vi "Begin.vi"() -> (0 "error out":errorcluster)   [LabVIEW 2013]
doc: "Called before other user functions, this VI is expected to open initial I/O refnums, load in file data, and do all program initialization. Notice that the <B>error out</B> terminal is simply used for data flow. Wiring it to other structures or subVIs ensures that this VI runs first."
uses:
  <vilib>/Rock Robotics/WPI/DriverStation/WPI_DriverStationRobotMode2.ctl
  <vilib>/Rock Robotics/WPI/Solenoid/WPI_SolenoidChannel.ctl
  <vilib>/Rock Robotics/WPI/SafetyOutput/WPI_SafetyOutputConfigMenu.ctl
  <vilib>/Rock Robotics/SystemInterfaces/DIO/FPGA_DIOChannel.ctl
  <vilib>/Rock Robotics/SystemInterfaces/DIO/FPGA_DIORelayChannel.ctl
  <vilib>/Rock Robotics/SystemInterfaces/AI/FPGA_AIGyroChannel.ctl
  <vilib>/Rock Robotics/SystemInterfaces/DIO/FPGA_DIOPWMChannel.ctl
  <vilib>/Rock Robotics/WPI/Joystick/WPI_JoystickDeviceEnum.ctl
  Robot Global Data.vi
  <vilib>/Rock Robotics/WPI/Solenoid/WPI_SolenoidOpenDouble.vi
  <vilib>/Rock Robotics/WPI/Counter/WPI_CounterDigitalInputToDigitalSource.vi
  <vilib>/Rock Robotics/WPI/MotorControl/WPI_MotorControlOpen Talon.vi
  <vilib>/Rock Robotics/WPI/Counter/WPI_CounterOpen Semi Period Mode.vi
  Auto Pickup Global.vi
  <vilib>/Rock Robotics/WPI/Compressor/WPI_CompressorGetSetRefNum.vi
  <vilib>/Rock Robotics/WPI/Relay/WPI_RelayDirection.ctl
  <vilib>/Rock Robotics/WPI/RobotDrive/WPI_RobotDriveOpen4MotorWithCANJaguar.vi
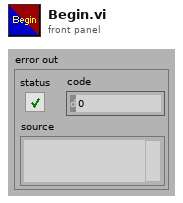
[diagram p1: front panel]
types:
  T1 = typedef "FPGA_DIOChannel.ctl" = enum8{"DIO 1", "DIO 2", "DIO 3", "DIO 4", "DIO 5", "DIO 6", "DIO 7", "DIO 8", "DIO 9", "DIO 10", "DIO 11", "DIO 12", "DIO 13", "DIO 14", "Invalid"}
  T2 = typedef "FPGA_DIOPWMChannel.ctl" = enum8{"PWM 1", "PWM 2", "PWM 3", "PWM 4", "PWM 5", "PWM 6", "PWM 7", "PWM 8", "PWM 9", "PWM 10", "Invalid"}
  T3 = typedef "WPI_JoystickDeviceEnum.ctl" = enum16{"USB 1", "USB 2", "USB 3", "USB 4", "Kinect 1", "Kinect 2"}
  T4 = typedef "WPI_SafetyOutputConfigMenu.ctl" = enum16{"Enable", "Disable"}
  T5 = typedef "FPGA_AIGyroChannel.ctl" = enum8{"AI 1", "AI 2", "Invalid"}
  T6 = typedef "FPGA_DIORelayChannel.ctl" = enum8{"Relay 1", "Relay 2", "Relay 3", "Relay 4", "Relay 5", "Relay 6", "Relay 7", "Relay 8", "Invalid"}
  T7 = typedef "WPI_SolenoidChannel.ctl" = enum8{"Solenoid 1", "Solenoid 2", "Solenoid 3", "Solenoid 4", "Solenoid 5", "Solenoid 6", "Solenoid 7", "Solenoid 8", "Invalid"}
  T8 = typedef "WPI_DriverStationRobotMode2.ctl" = enum16{"Autonomous Disabled", "Autonomous Enabled", "Teleop Disabled", "Teleop Enabled", "Timeout", "Finish", "Test Disabled", "Test Enabled"}
  T9 = typedef "WPI_RobotDriveDevRef.ctl" = cluster{"DevStatus":errorcluster, "Motors[]":T10[], "Square Inputs":bool, "Max Output":dbl, "Isochronous":bool}
  T10 = typedef "WPI_MotorControlDeviceRef.ctl" = cluster{"DeviceStatus":errorcluster, "Type":enum16{"PWM", "CAN"}, "PWM":cluster{"Digital Module":T11, "PWM Channel":T2, "DeadBand":T12}, "CAN":cluster{"Device Number":u8, "Control Mode":T13, "Semaphore":T14, "Max Vout":dbl}, "Invert":bool, "TransformRef":T15, "InvTransformRef":T15}
  T11 = typedef "FPGA_TypedefDigitalModule.ctl" = enum16{"Digital Module 1", "Digital Module 2"}
  T12 = typedef "WPI_PWMDeadband.ctl" = cluster{"Name":string, "maxPositivePwm":i32, "minPositivePwm":i32, "centerPwm":i32, "maxNegativePwm":i32, "minNegativePwm":i32, "angularRange":u16}
  T13 = typedef "WPI_CANJaguar_ControlMode.ctl" = enum8{"Percent VBus", "Current", "Speed", "Position", "Voltage"}
  T14 = typedef "Semaphore RefNum" = refnum<k1>
  T15 = typedef "WPI_PWMTransform_ConPane.ctl" = refnum<vi>
  T16 = typedef "WPI_DigitalInputDevRef.ctl" = cluster{"DevStatus":errorcluster, "DIO Channel":T1, "Digital Module":T11}
  T17 = typedef "FPGA_CounterEncoderSourceConvertionLVSourceType.ctl" = cluster{"DevStatus":errorcluster, "AnalogTriggerMode?":bool, "DigitalMode":cluster{"Digital Module":T11, "DIO Channel":T18}, "AnalogTriggerMode":cluster{"AnalogTriggerIndex":T19, "OutputType":T20}}
  T18 = typedef "FPGA_DIODigitalSourceChannel.ctl" = enum8{"DIO 1", "DIO 2", "DIO 3", "DIO 4", "DIO 5", "DIO 6", "DIO 7", "DIO 8", "DIO 9", "DIO 10", "DIO 11", "DIO 12", "DIO 13", "DIO 14", "Disabled"}
  T19 = typedef "FPGA_AnalogTriggerIndex.ctl" = enum8{"Trig 0", "Trig 1", "Trig 2", "Trig 3", "Trig 4", "Trig 5", "Trig 6", "Trig 7", "Invalid"}
  T20 = typedef "FPGA_AnalogTriggerOutType.ctl" = enum16{"InWindow", "TriggerState", "Rising", "Falling"}
  T21 = typedef "WPI_CompressorDevRef.ctl" = cluster{"DevStatus":errorcluster, "DigitalInputDevRef":T16, "RelayDevRef":T22}
  T22 = typedef "WPI_RelayDevRef.ctl" = cluster{"DevStatus":errorcluster, "Relay Channel":T6, "Digital Module":T11, "Relay Direction":T23}
  T23 = typedef "WPI_RelayDirection.ctl" = enum16{"Both directions", "Forward only", "Reverse only"}
  T24 = typedef "WPI_EncoderDevRef.ctl" = cluster{"DevStatus":errorcluster, "EncoderIndex":T25, "CounterIndex":T26, "DistancePerCount":dbl, "Decoding Type":T27}
  T25 = typedef "FPGA_EncoderIdx.ctl" = enum8{"Enc 0", "Enc 1", "Enc 2", "Enc 3", "Invalid"}
  T26 = typedef "FPGA_CounterCtrSystemIndex.ctl" = enum8{"Ctr 0", "Ctr 1", "Ctr 2", "Ctr 3", "Ctr 4", "Ctr 5", "Ctr 6", "Ctr 7", "Invalid"}
  T27 = typedef "WPI_EncoderType.ctl" = enum16{"1x", "2x", "4x"}
  T28 = typedef "WPI_CounterDevRef.ctl" = cluster{"DevStatus":errorcluster, "CntIndex":T26}
  T29 = typedef "WPI_GyroDevRef.ctl" = cluster{"DevStatus":errorcluster, "Analog Module":T30, "Analog Channel":T31, "Offset":dbl, "Gain (VoltsPerDegree/Second)":dbl}
  T30 = typedef "FPGA_TypedefAnalogModule.ctl" = enum16{"Analog Module 1", "Analog Module 2"}
  T31 = typedef "FPGA_AIChannel.ctl" = enum8{"AI 1", "AI 2", "AI 3", "AI 4", "AI 5", "AI 6", "AI 7", "AI 8", "Invalid"}
  T32 = typedef "WPI_I2CDevRef.ctl" = cluster{"DevStatus":errorcluster, "Digital Module":T11, "Device Address":u8}
  T33 = typedef "WPI_JoystickDevRef.ctl" = cluster{"Device":T3}
  T34 = typedef "LEDStripRef.ctl" = cluster{"PWM Rate (Hz)":sgl, "Max Duty Cycle":sgl, "DigitalOutputRed":T35, "DigitalOutputGreen":T35, "DigitalOutputBlue":T35, "DevStatus":errorcluster}
  T35 = typedef "WPI_DigitalOutputDevRef.ctl" = cluster{"Digital Module":T11, "DIO Channel":T1, "DevStatus":errorcluster}
  T36 = typedef "WPI_SolenoidDevRef.ctl" = cluster{"DevStatus":errorcluster, "Solenoid Module":T37, "Forward Solenoid Channel":T7, "Reverse Solenoid Channel":T7}
  T37 = typedef "FPGA_TypedefSolenoidModule.ctl" = enum16{"Solenoid Module 1", "Solenoid Module 2"}
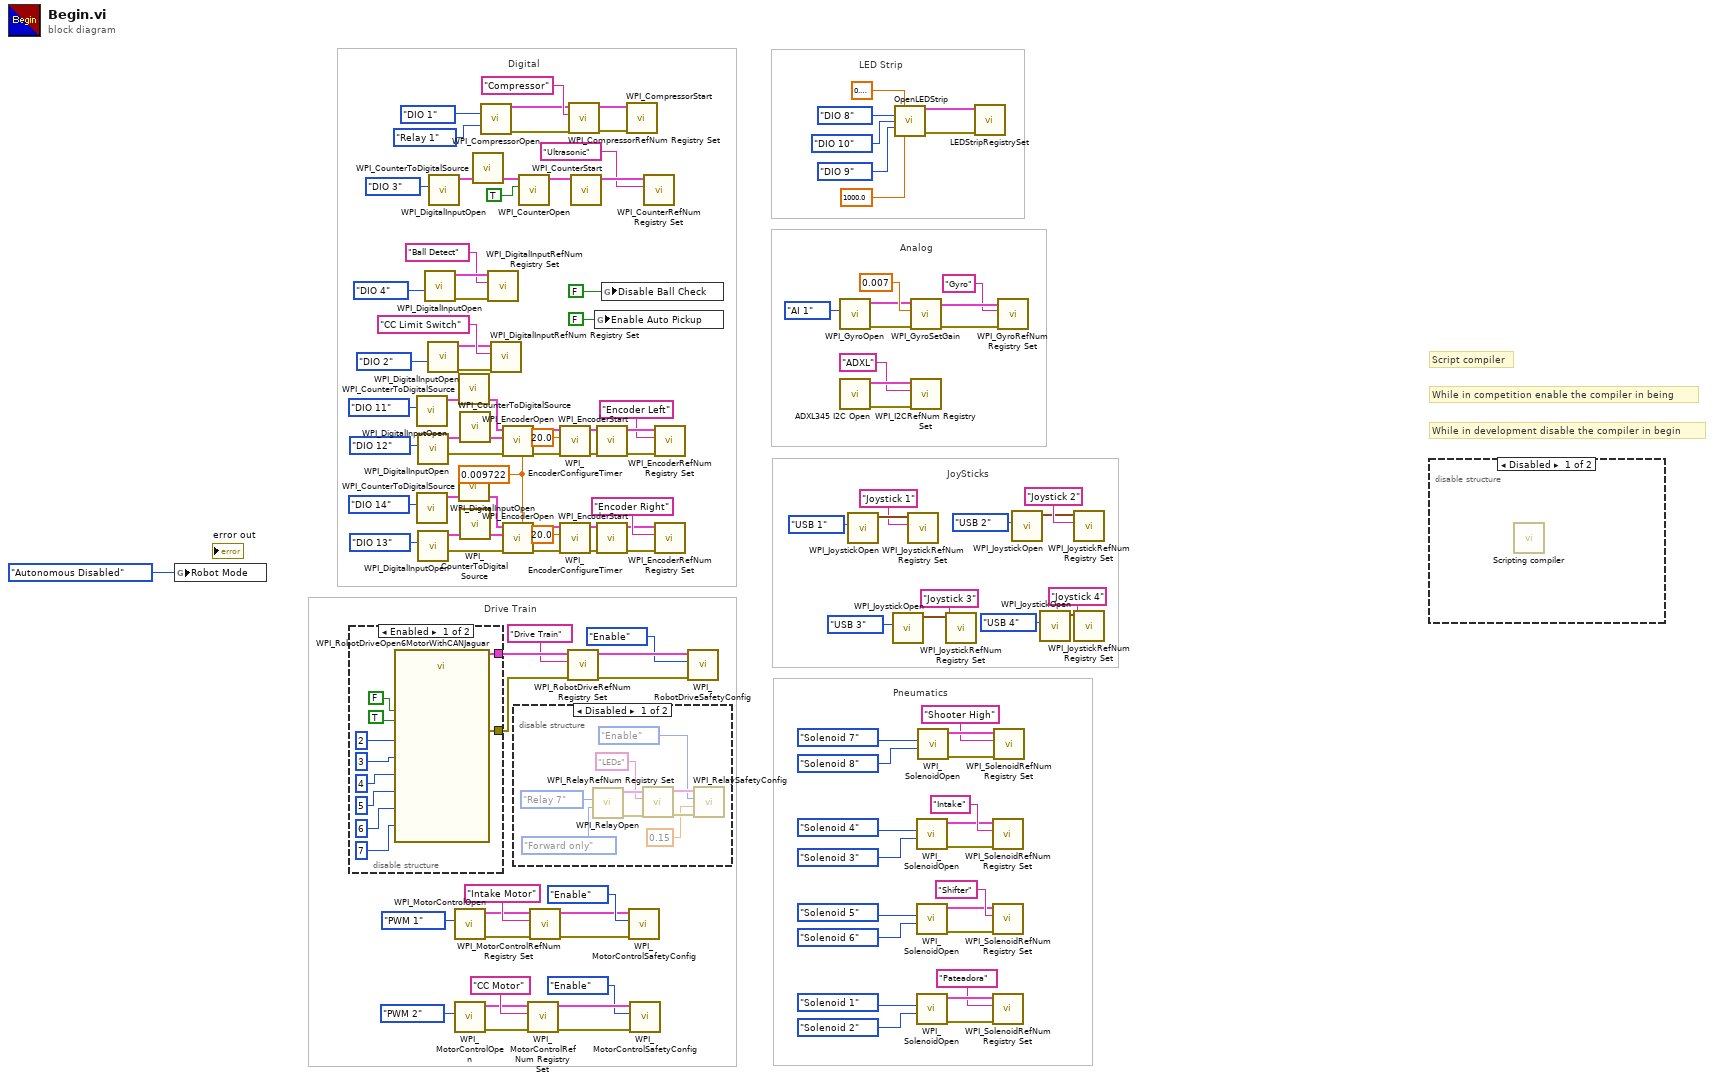
[diagram p0: block diagram]
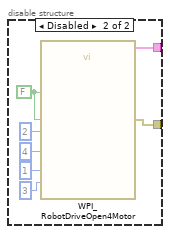
[diagram p3: hidden frame]
diagram:
  w11 = 0.009722 ("DistancePerCount")
  # "LED Strip"
  # "While in development disable the compiler in begin"
  # "While in competition enable the compiler in being"
  # "Script compiler"
  # "JoySticks"
  # "Analog"
  # "Digital"
  # "Drive Train"
  # "Pneumatics"
  n1 = global write "Robot Global Data.vi" "Robot Mode"(WPI_DriverStationRobotMode2."Autonomous Disabled" ("Robot Mode")) -> ()
  n2 = disable-structure shown="Enabled" {
    disable-tunnel: [w133 w142] -> w107
    disable-tunnel: [w132 w136] -> w100
    frame Enabled {
      n3 = call <vilib>:"WPI_RobotDriveOpen6MotorWithCANJaguar.vi"("Rear Left Motor"=u8 4, "Rear Right Motor"=u8 7 ("Mid Right Motor"), "Front Right Motor"=u8 5 ("Rear Right Motor"), "Front Left Motor"=u8 2, "Mid Left Motor"=u8 3 ("Front Right Motor"), "Mid Right Motor"=u8 6 ("Mid Left Motor"), "Left Motors Inverted"=FALSE, "Right Motors Inverted"=TRUE) -> ("RobotDriveDevRef"=w133:T9, "error out"=w132:errorcluster)  [unwired: 10 in]
    }
    frame Disabled {
      w137 = FALSE ("Front Left Motor Inverted")
      n4 = call-poly <vilib>:"WPI_RobotDriveOpen4Motor.vi"("Rear Left Motor"=u8 4, "Rear Left Motor Inverted"=w137, "Rear Right Motor"=u8 3, "Front Left Motor"=u8 2, "Front Right Motor"=u8 1, "Front Left Motor Inverted"=w137) -> ("RobotDriveDevRef"=w142:T9, "error out"=w136:errorcluster)  [unwired: 8 in]
    }
  }
  n5 = call <vilib>:"WPI_DigitalInputOpen.vi"("DIO Channel"=FPGA_DIOChannel."DIO 11") -> ("DigitalInputDevRef"=w99:T16)  [unwired: 2 in, 8 out]
  n6 = call <vilib>:"WPI_DigitalInputOpen.vi"("DIO Channel"=FPGA_DIOChannel."DIO 14") -> ("DigitalInputDevRef"=w14:T16)  [unwired: 2 in, 8 out]
  n7 = call <vilib>:"WPI_DigitalInputOpen.vi"("DIO Channel"=FPGA_DIOChannel."DIO 12") -> ("error out"=w85:errorcluster, "DigitalInputDevRef"=w90:T16)  [unwired: 2 in, 7 out]
  n8 = call <vilib>:"WPI_DigitalInputOpen.vi"("DIO Channel"=FPGA_DIOChannel."DIO 13") -> ("error out"=w28:errorcluster, "DigitalInputDevRef"=w23:T16)  [unwired: 2 in, 7 out]
  n9 = call <vilib>:"WPI_DigitalInputOpen.vi"("DIO Channel"=FPGA_DIOChannel."DIO 4") -> ("error out"=w29:errorcluster, "DigitalInputDevRef"=w32:T16)  [unwired: 9 in]
  n10 = call <vilib>:"WPI_DigitalInputOpen.vi"("DIO Channel"=FPGA_DIOChannel."DIO 2") -> ("error out"=w81:errorcluster, "DigitalInputDevRef"=w82:T16)  [unwired: 9 in]
  n11 = call <vilib>:"WPI_DigitalInputOpen.vi"("DIO Channel"=FPGA_DIOChannel."DIO 3") -> ("DigitalInputDevRef"=w43:T16)  [unwired: 2 in, 8 out]
  n12 = call-poly <vilib>:"WPI_MotorControlOpen.vi"("PWM Channel"=FPGA_DIOPWMChannel."PWM 1") -> ("error out"=w70:errorcluster, "MotorControlDeviceRef"=w62:T10)  [unwired: 9 in]
  n13 = call-poly <vilib>:"WPI_MotorControlOpen.vi"("PWM Channel"=FPGA_DIOPWMChannel."PWM 2") -> ("error out"=w67:errorcluster, "MotorControlDeviceRef"=w61:T10)  [unwired: 9 in]
  n14 = call-poly <vilib>:"WPI_CounterToDigitalSource.vi"("DigitalInputDevRef"=w99) -> ("Digital Source"=w98:T17)  [unwired: 6 out]
  n15 = call-poly <vilib>:"WPI_CounterToDigitalSource.vi"("DigitalInputDevRef"=w14) -> ("Digital Source"=w15:T17)  [unwired: 6 out]
  n16 = call-poly <vilib>:"WPI_CounterToDigitalSource.vi"("DigitalInputDevRef"=w90) -> ("Digital Source"=w89:T17)  [unwired: 6 out]
  n17 = call-poly <vilib>:"WPI_CounterToDigitalSource.vi"("DigitalInputDevRef"=w23) -> ("Digital Source"=w24:T17)  [unwired: 6 out]
  n18 = call-poly <vilib>:"WPI_CounterToDigitalSource.vi"("DigitalInputDevRef"=w43) -> ("Digital Source"=w41:T17)  [unwired: 6 in]
  n19 = call <vilib>:"WPI_CompressorOpen.vi"("Pressure Switch DIO Channel"=FPGA_DIOChannel."DIO 1", "Relay Channel"=FPGA_DIORelayChannel."Relay 1") -> ("CompressorDevRef"=w36:T21, "error out"=w37:errorcluster)  [unwired: 12 in]
  n20 = call <vilib>:"WPI_DigitalInputRefNum Registry Set.vi"("error in (no error)"=w29, "refnum name"="Ball Detect", "DigitalInputDevRef"=w32) -> ()  [unwired: 7 in, 2 out]
  n21 = call <vilib>:"WPI_DigitalInputRefNum Registry Set.vi"("error in (no error)"=w81, "refnum name"="CC Limit Switch", "DigitalInputDevRef"=w82) -> ()  [unwired: 7 in, 2 out]
  n22 = call <vilib>:"WPI_EncoderOpen.vi"("DistancePerCount"=w11, "error in (no error)"=w85, "BSource"=w89, "ASource"=w98) -> ("error out"=w88:errorcluster, "EncoderDevRef"=w96:T24)  [unwired: 4 in, 2 out]
  n23 = call <vilib>:"WPI_EncoderOpen.vi"("DistancePerCount"=w11, "error in (no error)"=w28, "BSource"=w24, "ASource"=w15) -> ("error out"=w25:errorcluster, "EncoderDevRef"=w17:T24)  [unwired: 4 in, 2 out]
  n24 = disable-structure shown="Disabled" {
    frame Disabled {
      n25 = call <vilib>:"WPI_RelayOpen.vi"("Relay Direction"=WPI_RelayDirection."Forward only", "Relay Channel"=FPGA_DIORelayChannel."Relay 7") -> ("error out"=w149:errorcluster, "RelayDevRef"=w148:T22)  [unwired: 8 in]
      n26 = call <vilib>:"WPI_RelayRefNum Registry Set.vi"("error in (no error)"=w149, "refnum name"="LEDs", "RelayDevRef"=w148) -> ("error out"=w146:errorcluster, "RelayDevRef"=w145:T22)  [unwired: 7 in]
      n27 = call <vilib>:"WPI_RelaySafetyConfig.vi"("error in (no error)"=w146, "timeout (s)"=0.15, "mode"=WPI_SafetyOutputConfigMenu."Enable", "RelayDevRef"=w145) -> ()  [unwired: 6 in, 2 out]
    }
    frame Enabled {
    }
  }
  n28 = call-poly <vilib>:"WPI_CounterOpen.vi"("High Pulse (T)"=TRUE, "Source"=w41) -> ("CounterDevRef"=w42:T28)  [unwired: 8 in, 1 out]
  n29 = call <vilib>:"WPI_MotorControlRefNum Registry Set.vi"("error in (no error)"=w67, "refnum name"="CC Motor", "MotorControlDevRef"=w61) -> ("error out"=w64:errorcluster, "MotorControlDevRef"=w68:T10)  [unwired: 7 in]
  n30 = call <vilib>:"WPI_MotorControlRefNum Registry Set.vi"("error in (no error)"=w70, "refnum name"="Intake Motor", "MotorControlDevRef"=w62) -> ("error out"=w73:errorcluster, "MotorControlDevRef"=w69:T10)  [unwired: 7 in]
  n31 = call <vilib>:"WPI_EncoderConfigureTimer.vi"("error in (no error)"=w88, "Minimum Rate"=20.0, "EncoderDevRef"=w96) -> ("error out"=w87:errorcluster, "EncoderDevRef"=w97:T24)  [unwired: 1 in, 6 out]
  n32 = call <vilib>:"WPI_EncoderConfigureTimer.vi"("error in (no error)"=w25, "Minimum Rate"=20.0, "EncoderDevRef"=w17) -> ("error out"=w26:errorcluster, "EncoderDevRef"=w16:T24)  [unwired: 1 in, 6 out]
  n33 = call <vilib>:"WPI_RobotDriveRefNum Registry Set.vi"("error in (no error)"=w100, "refnum name"="Drive Train", "RobotDriveDevRef"=w107) -> ("error out"=w101:errorcluster, "RobotDriveDevRef"=w108:T9)  [unwired: 7 out]
  n34 = call <vilib>:"WPI_CompressorRefNum Registry Set.vi"("error in (no error)"=w37, "refnum name"="Compressor", "CompressorDevRef"=w36) -> ("error out"=w35:errorcluster, "CompressorDevRef"=w34:T21)  [unwired: 7 in]
  n35 = call <vilib>:"WPI_CounterStart.vi"("CounterDevRef in"=w42) -> ("CounterDevRef out"=w39:T28)  [unwired: 9 in, 1 out]
  n36 = global write "Auto Pickup Global.vi" "Enable Auto Pickup"(FALSE ("Enable Auto Pickup")) -> ()
  n37 = call <vilib>:"WPI_EncoderStart.vi"("error in (no error)"=w87, "EncoderDevRef"=w97) -> ("error out"=w86:errorcluster, "EncoderDevRef"=w94:T24)  [unwired: 8 out]
  n38 = call <vilib>:"WPI_EncoderStart.vi"("error in (no error)"=w26, "EncoderDevRef"=w16) -> ("error out"=w27:errorcluster, "EncoderDevRef"=w19:T24)  [unwired: 8 out]
  n39 = global write "Robot Global Data.vi" "Disable Ball Check"(FALSE ("Disable Ball Check")) -> ()
  n40 = call <vilib>:"WPI_CompressorStart.vi"("error in (no error)"=w35, "CompressorDevRef"=w34) -> ()  [unwired: 8 in, 2 out]
  n41 = call <vilib>:"WPI_MotorControlSafetyConfig.vi"("error in (no error)"=w73, "mode"=WPI_SafetyOutputConfigMenu."Enable", "MotorControlDevRef"=w69) -> ()  [unwired: 7 in, 2 out]
  n42 = call <vilib>:"WPI_MotorControlSafetyConfig.vi"("error in (no error)"=w64, "mode"=WPI_SafetyOutputConfigMenu."Enable", "MotorControlDevRef"=w68) -> ()  [unwired: 7 in, 2 out]
  n43 = call <vilib>:"WPI_CounterRefNum Registry Set.vi"("refnum name"="Ultrasonic", "CounterDevRef"=w39) -> ()  [unwired: 8 in, 2 out]
  n44 = call <vilib>:"WPI_EncoderRefNum Registry Set.vi"("error in (no error)"=w86, "refnum name"="Encoder Left", "EncoderDevRef"=w94) -> ()  [unwired: 7 in, 2 out]
  n45 = call <vilib>:"WPI_EncoderRefNum Registry Set.vi"("error in (no error)"=w27, "refnum name"="Encoder Right", "EncoderDevRef"=w19) -> ()  [unwired: 7 in, 2 out]
  n46 = call <vilib>:"WPI_RobotDriveSafetyConfig.vi"("error in (no error)"=w101, "mode"=WPI_SafetyOutputConfigMenu."Enable", "RobotDriveDevRef"=w108) -> ()  [unwired: 7 in, 2 out]
  n47 = call <vilib>:"WPI_GyroOpen.vi"("Analog Channel"=FPGA_AIGyroChannel."AI 1") -> ("error out"=w75:errorcluster, "GyroDevRef"=w78:T29)  [unwired: 8 in, 1 out]
  n48 = call "ADXL345 I2C Open.vi"() -> ("error out"=w1:errorcluster, "I2CDevRef"=w3:T32)  [unwired: 10 in]
  n49 = call <vilib>:"WPI_JoystickOpen.vi"("JoystickDevice"=WPI_JoystickDeviceEnum."USB 1") -> ("JoystickDevRef"=w59:T33)  [unwired: 10 in]
  n50 = call <vilib>:"WPI_JoystickOpen.vi"("JoystickDevice"=WPI_JoystickDeviceEnum."USB 3") -> ("JoystickDevRef"=w53:T33)  [unwired: 10 in]
  n51 = call "OpenLEDStrip.vi"("Max Duty Cycle (1)"=sgl 0.2 ("Max Duty Cycle"), "DIO Channel Red"=FPGA_DIOChannel."DIO 8" ("DIO Channel"), "DIO Channel Green"=FPGA_DIOChannel."DIO 10" ("DIO Channel"), "DIO Channel Blue"=FPGA_DIOChannel."DIO 9" ("DIO Channel"), "PWM Rate (Hz)"=sgl 1000.0) -> ("LEDStripRef"=w7:T34, "error out"=w6:errorcluster)  [unwired: 9 in]
  n52 = call <vilib>:"WPI_JoystickRefNum Registry Set.vi"("refnum name"="Joystick 1", "JoystickDevRef"=w59) -> ()  [unwired: 8 in, 2 out]
  n53 = call <vilib>:"WPI_GyroSetGain.vi"("error in (no error)"=w75, "Gain (VoltsPerDegree/Second)"=0.007, "GyroDevRef"=w78) -> ("error out"=w74:errorcluster, "GyroDevRef"=w80:T29)  [unwired: 7 in]
  n54 = call <vilib>:"WPI_I2CRefNum Registry Set.vi"("error in (no error)"=w1, "refnum name"="ADXL", "I2CDevRef"=w3) -> ()  [unwired: 7 in, 2 out]
  n55 = call-poly <vilib>:"WPI_SolenoidOpen.vi"("Reverse Solenoid Channel"=WPI_SolenoidChannel."Solenoid 3" ("Solenoid Channel"), "Forward Solenoid Channel"=WPI_SolenoidChannel."Solenoid 4" ("Solenoid Channel")) -> ("error out"=w118:errorcluster, "SolenoidDevRef"=w119:T36)  [unwired: 8 in]
  n56 = call-poly <vilib>:"WPI_SolenoidOpen.vi"("Reverse Solenoid Channel"=WPI_SolenoidChannel."Solenoid 6" ("Solenoid Channel"), "Forward Solenoid Channel"=WPI_SolenoidChannel."Solenoid 5" ("Solenoid Channel")) -> ("error out"=w110:errorcluster, "SolenoidDevRef"=w111:T36)  [unwired: 8 in]
  n57 = call-poly <vilib>:"WPI_SolenoidOpen.vi"("Reverse Solenoid Channel"=WPI_SolenoidChannel."Solenoid 2" ("Solenoid Channel"), "Forward Solenoid Channel"=WPI_SolenoidChannel."Solenoid 1" ("Solenoid Channel")) -> ("error out"=w115:errorcluster, "SolenoidDevRef"=w114:T36)  [unwired: 8 in]
  n58 = call-poly <vilib>:"WPI_SolenoidOpen.vi"("Reverse Solenoid Channel"=WPI_SolenoidChannel."Solenoid 8" ("Solenoid Channel"), "Forward Solenoid Channel"=WPI_SolenoidChannel."Solenoid 7" ("Solenoid Channel")) -> ("error out"=w123:errorcluster, "SolenoidDevRef"=w122:T36)  [unwired: 8 in]
  n59 = call <vilib>:"WPI_JoystickRefNum Registry Set.vi"("refnum name"="Joystick 3", "JoystickDevRef"=w53) -> ()  [unwired: 8 in, 2 out]
  n60 = call "LEDStripRegistrySet.vi"("error in"=w6, "LEDStripRef"=w7) -> ()  [unwired: 8 in, 2 out]
  n61 = call <vilib>:"WPI_SolenoidRefNum Registry Set.vi"("error in (no error)"=w118, "refnum name"="Intake", "SolenoidDevRef"=w119) -> ()  [unwired: 7 in, 2 out]
  n62 = call <vilib>:"WPI_SolenoidRefNum Registry Set.vi"("error in (no error)"=w110, "refnum name"="Shifter", "SolenoidDevRef"=w111) -> ()  [unwired: 7 in, 2 out]
  n63 = call <vilib>:"WPI_SolenoidRefNum Registry Set.vi"("error in (no error)"=w115, "refnum name"="Pateadora", "SolenoidDevRef"=w114) -> ()  [unwired: 7 in, 2 out]
  n64 = call <vilib>:"WPI_SolenoidRefNum Registry Set.vi"("error in (no error)"=w123, "refnum name"="Shooter High", "SolenoidDevRef"=w122) -> ()  [unwired: 7 in, 2 out]
  n65 = call <vilib>:"WPI_GyroRefNum Registry Set.vi"("error in (no error)"=w74, "refnum name"="Gyro", "GyroDevRef"=w80) -> ()  [unwired: 7 in, 2 out]
  n66 = call <vilib>:"WPI_JoystickOpen.vi"("JoystickDevice"=WPI_JoystickDeviceEnum."USB 2") -> ("JoystickDevRef"=w56:T33)  [unwired: 10 in]
  n67 = call <vilib>:"WPI_JoystickOpen.vi"("JoystickDevice"=WPI_JoystickDeviceEnum."USB 4") -> ("JoystickDevRef"=w50:T33)  [unwired: 10 in]
  n68 = call <vilib>:"WPI_JoystickRefNum Registry Set.vi"("refnum name"="Joystick 2", "JoystickDevRef"=w56) -> ()  [unwired: 8 in, 2 out]
  n69 = call <vilib>:"WPI_JoystickRefNum Registry Set.vi"("refnum name"="Joystick 4", "JoystickDevRef"=w50) -> ()  [unwired: 8 in, 2 out]
  n70 = disable-structure shown="Disabled" {
    frame Disabled {
      n71 = call "Scripting compiler.vi"() -> ()  [unwired: 12 in]
    }
    frame Enabled {
    }
  }
